vi "Read GSstatus.lvclass.vi"(8 "error in (no error)":errorcluster, 11 "GSserver in":refnum<class "GSserver.lvclass">) -> (0 "error out":errorcluster, 2 "GSstatus.lvclass":refnum<class "GSstatus.lvclass">, 3 "GSserver out":refnum<class "GSserver.lvclass">)   [LabVIEW 2018, in "GSserver.lvclass"]
uses:
  GSserver.lvclass
  GSstatus/GSstatus.lvclass
  GSserver.lvclass/GSserver.ctl
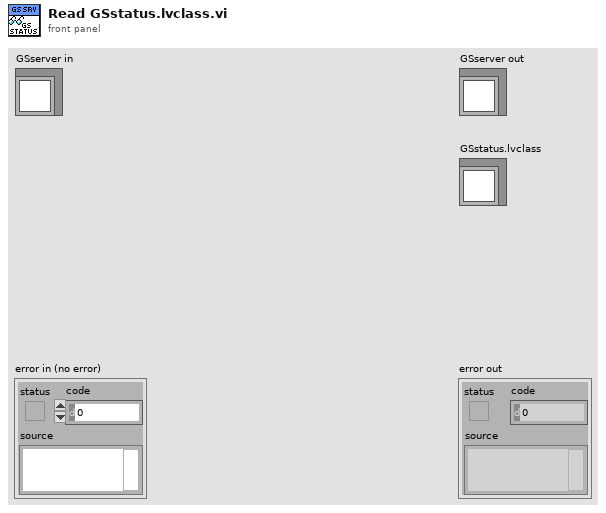
[diagram p1: front panel]
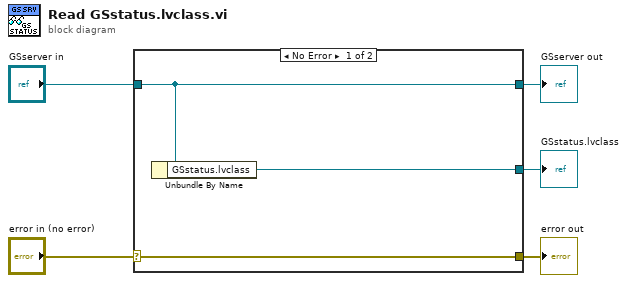
[diagram p0: block diagram]
diagram:
  n1 = case shown="No Error" "error in (no error)" {
    selector: "error in (no error)" -> [w8 w9]
    tunnel: [w8 w9] -> w4
    tunnel: [w7 w10] -> w2
    tunnel: "GSserver in" -> [w7 w10]
    tunnel: [w6 _] -> w1
    frame No Error {
      n2 = Unbundle By Name(w7) -> ("GSstatus.lvclass"=w6:refnum<class "GSstatus.lvclass">)
    }
    frame Error {
    }
  }
  "error out" <- w4
  "GSserver out" <- w2
  "GSstatus.lvclass" <- w1
